vi "Grava LOG T-RH-N.vi"(8 "N2 flow":sgl format="%#.3g", 9 "N2 setpoint":sgl, 10 "Humidity":sgl, 11 "Temperature":sgl) -> (0 "error out":errorcluster)   [LabVIEW 2015, in "VIPM2.lvlib"]
doc: "LOG: temperatura, humitat i nitrogen.\nFile path: C:\\VIP Module x2\\Files\\T-RH-N.log\nSi no existeix l'arxiu, el crea.\nAfegeix els registres al final de l'arxiu.\nSi és 1a execució o canvi de dia, afegeix una capçalera."
uses:
  VIPM2.lvlib
panel:
  # "LOG: temperatura, humitat i nitrogen"
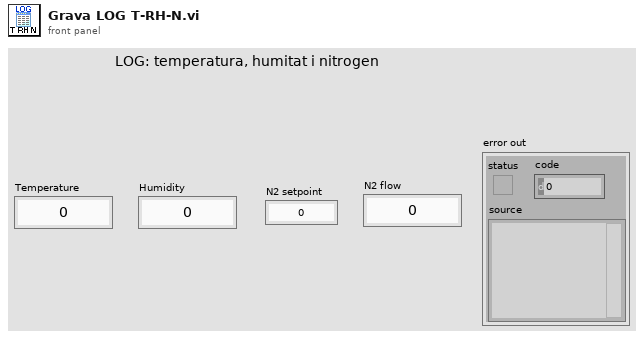
[diagram p1: front panel]
types:
  T1 = enum16{"open", "replace", "create", "open or create", "replace or create", "replace or create with confirmation"}
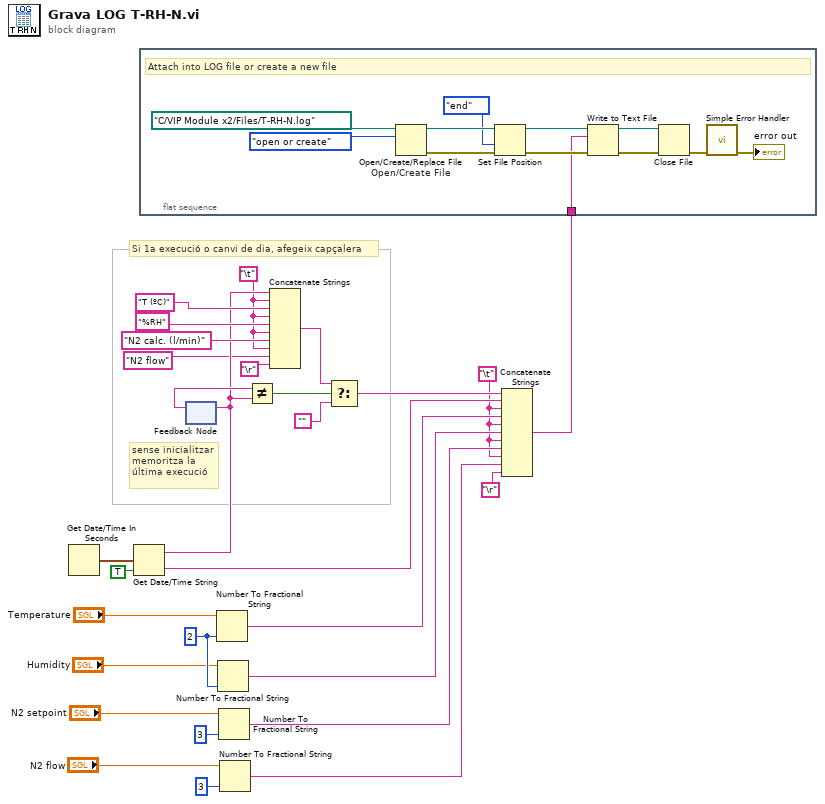
[diagram p0: block diagram]
diagram:
  w16 = i16 2 ("precision (6)")
  w7 = "\t"
  w4 = "\t"
  # "sense inicialitzar\nmemoritza la\núltima execució"
  # "Si 1a execució o canvi de dia, afegeix capçalera"
  n1 = Get Date/Time In Seconds() -> (seconds since 1Jan1904=w29:timestamp)
  n2 = Get Date/Time String(seconds (now)=w29, want seconds? (F)=TRUE) -> (date string=w9:string, time string=w22:string)  [unwired: 1 in]
  n3 = flat-sequence {
    tunnel: w21 -> [w31]
    frame #0 {
      # "Attach into LOG file or create a new file"
      n4 = Open/Create/Replace File "Open/Create File"(file path (use dialog)=path "C:/VIP Module x2/Files/T-RH-N.log", operation (0:open)=T1."open or create") -> (refnum out=w39:refnum<file>, error out=w38:errorcluster)  [unwired: 4 in, 1 out]
      n5 = Set File Position(refnum=w39, from (0:start)=enum16{"start", "end", "current"}."end", error in=w38) -> (refnum out=w36:refnum<file>, error out=w35:errorcluster)  [unwired: 1 in]
      n6 = Write to Text File(file (use dialog)=w36, text=w31, error in=w35) -> (refnum out=w34:refnum<file>, error out=w33:errorcluster)  [unwired: 1 in, 1 out]
      n7 = Close File(refnum=w34, error in=w33) -> (error out=w32:errorcluster)  [unwired: 1 out]
      n8 = call <vilib>:"Simple Error Handler.vi"("error in (no error)"=w32) -> ("error out"=→"error out":errorcluster)  [unwired: 4 in, 4 out]
    }
  }
  n9 = feedback-in #1(w9) -> ()
  n10 = feedback #1() -> (w27:string)  [unwired: 1 in]
  n11 = Number To Fractional String(number="Temperature", precision (6)=w16) -> (F-format string=w14:string)  [unwired: 2 in]
  n12 = Number To Fractional String(number="Humidity", precision (6)=w16) -> (F-format string=w13:string)  [unwired: 2 in]
  n13 = Number To Fractional String(number="N2 setpoint", precision (6)=i16 3) -> (F-format string=w19:string)  [unwired: 2 in]
  n14 = Number To Fractional String(number="N2 flow", precision (6)=i16 3) -> (F-format string=w1:string)  [unwired: 2 in]
  n15 = Not Equal?(x=w27, y=w9) -> (x != y?=w24:bool)
  n16 = Concatenate Strings "Concatenate Strings"(w9, w7, "T (ºC)" ("string"), w7, "%RH" ("string"), w7, "N2 calc. (l/min)" ("string"), w7, "N2 flow" ("string"), "\r") -> (w25:string)
  n17 = Select(t=w25, s=w24, f="") -> (s? t:f=w23:string)
  n18 = Concatenate Strings "Concatenate Strings"(w23, w22, w4, w14, w4, w13, w4, w19, w4, w1, "\r") -> (w21:string)
